vi "Coded Eval Parsed Formula String.vi"(2 "error in (no error)":errorcluster, 3 "Parsed Formula":cluster{"Table":i32[][], "Y Values":dbl[]} {"Y Values" format="%0.2f"}, 4 "Variables":i32[](array[numeric]), 5 "X Values":dbl[](array[numeric]) format="%0.2f") -> (0 "error out":errorcluster, 1 "y value":dbl format="%0.2f")   [LabVIEW 2017, in "NI_Gmath.lvlib"]
uses:
  <vilib>/gmath/NI_Gmath.lvlib
panel:
  # "Example:\n\n See Parse Formula String.vi!"
  # "operator"
  # "register1"
  # "register2"
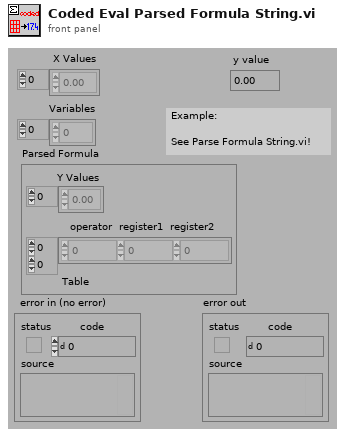
[diagram p1: front panel]
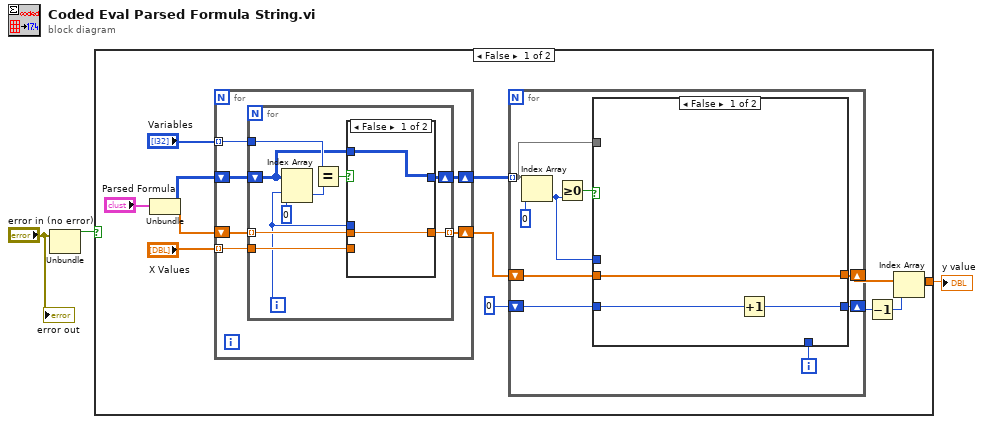
[diagram p0: block diagram]
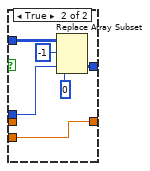
[diagram p2: hidden frame]
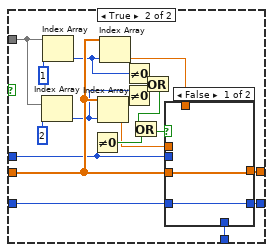
[diagram p3: hidden frame]
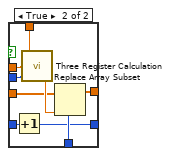
[diagram p4: hidden frame]
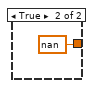
[diagram p5: hidden frame]
diagram:
  n1 = Unbundle("error in (no error)") -> ("status"=w2:bool)  [unwired: 2 out]
  n2 = case shown="False" w2 {
    tunnel: [w7 nan] -> w3
    frame False {
      n3 = Unbundle("Parsed Formula") -> ("Table"=w5:i32[][], "Y Values"=w4:dbl[])
      n4 = for {
        shift-right: [w16] -> w10
        shift-left: w5 -> [w17]
        tunnel: "Variables" -> [w21] mode=indexing
        shift-right: [w19] -> w12
        shift-left: w4 -> [w20]
        tunnel: "X Values" -> [w18] mode=indexing
        n5 = for {
          tunnel: w21 -> [w31]
          tunnel: w20 -> [w29] mode=indexing
          tunnel: [w28] -> w19 mode=indexing
          tunnel: w18 -> [w27]
          shift-right: [w22] -> w16
          shift-left: w17 -> [w23]
          i -> [w24]
          n6 = Index Array(array=w23, index (row)=w24, index (col)=0) -> (element=w25:i32)
          n7 = Equal?(x=w31, y=w25) -> (x = y?=w30:bool)
          n8 = case shown="False" w30 {
            tunnel: [w33 w39] -> w28
            tunnel: w29 -> [w33 _]
            tunnel: w27 -> [_ w39]
            tunnel: w23 -> [w32 w38]
            tunnel: [w32 w36] -> w22
            tunnel: w24 -> [_ w35]
            frame False {
            }
            frame True {
              n9 = Replace Array Subset(array=w38, new element=-1, index (row)=w35, index (col)=0) -> (w36:i32[][])
            }
          }
        }
      }
      n10 = for {
        tunnel: w10 -> [w45] mode=indexing
        shift-right: [w42] -> w11
        shift-left: w12 -> [w43]
        shift-right: [w40] -> w14
        shift-left: 0 -> [w41]
        i -> [w44]
        n11 = Index Array(array=w45, index=0) -> (element=w46:i32)
        n12 = Greater Or Equal To 0?(x=w46) -> (x >= 0?=w47:bool)
        n13 = case shown="False" w47 {
          tunnel: w46 -> [_ w61]
          tunnel: w45 -> [_ w67]
          tunnel: w44 -> [_ w66]
          tunnel: w43 -> [w51 w65]
          tunnel: [w51 w64] -> w42
          tunnel: w41 -> [w50 w53]
          tunnel: [w49 w52] -> w40
          frame False {
            n14 = Increment(x=w50) -> (x+1=w49:i32)
          }
          frame True {
            n15 = Index Array(array=w67, index=2) -> (element=w54:i32)
            n16 = Index Array(array=w67, index=1) -> (element=w55:i32)
            n17 = Not Equal To 0?(x=w61) -> (x != 0?=w59:bool)
            n18 = Index Array(array=w65, index=w54) -> (element=w56:dbl)
            n19 = Index Array(array=w65, index=w55) -> (element=w57:dbl)
            n20 = Not Equal To 0?(x=w55) -> (x != 0?=w62:bool)
            n21 = Not Equal To 0?(x=w54) -> (x != 0?=w63:bool)
            n22 = Or(x=w62, y=w63) -> (x .or. y?=w60:bool)
            n23 = Or(x=w60, y=w59) -> (x .or. y?=w58:bool)
            n24 = case shown="False" w58 {
              tunnel: [w71 w80] -> w64
              tunnel: w65 -> [w71 w78]
              tunnel: w66 -> [_ w77]
              tunnel: w56 -> [_ w76]
              tunnel: w57 -> [_ w75]
              tunnel: w61 -> [_ w74]
              tunnel: w53 -> [w70 w73]
              tunnel: [w70 w72] -> w52
              frame False {
              }
              frame True {
                n25 = Increment(x=w73) -> (x+1=w72:i32)
                n26 = call <vilib>:"Three Register Calculation.VI"("operation"=w74, "before last"=w76, "last"=w75) -> ("result"=w79:dbl)
                n27 = Replace Array Subset(array=w78, new element=w79, index=w77) -> (w80:dbl[])
              }
            }
          }
        }
      }
      n28 = Decrement(x=w14) -> (x-1=w15:i32)
      n29 = Index Array(array=w11, index=w15) -> (element=w7:dbl)
    }
    frame True {
    }
  }
  "y value" <- w3
  "error out" <- "error in (no error)"
